vi "BatteryCharge1.vi"() -> ()   [LabVIEW 2020]
uses:
  <instrlib>/NH Research Regenerative Test Series/Public/Configure/Output Safety.ctl
  <instrlib>/NH Research Regenerative Test Series/Public/Data/Read (Ave Current).vi
  <instrlib>/NH Research Regenerative Test Series/Public/Data/Low Level/Fetch (Ave Voltage).vi
  <instrlib>/NH Research Regenerative Test Series/Public/Data/Low Level/Fetch (Ave True Power).vi
  <instrlib>/NH Research Regenerative Test Series/NH Research Regenerative Test Series.lvlib
panel:
  in  "Output Safety":T1
  out "Current Compare":dbl
  in  "Current Cutoff":dbl
  out "Ave Current (A)":dbl
  out "Ave Voltage (V)":dbl
  out "Ave True Power (W)":dbl
  out "Status Byte Register":T2
  in  "Logical Instrument Number":u32=1
  in  "Charge Current":dbl format="%#.6g"
  in  "Charge Voltage":dbl format="%#.6g"
  in  "Battery Detect Voltage (0V)":dbl format="%#.6g"
  in  "VISA resource name":refnum<visa-resource-name>
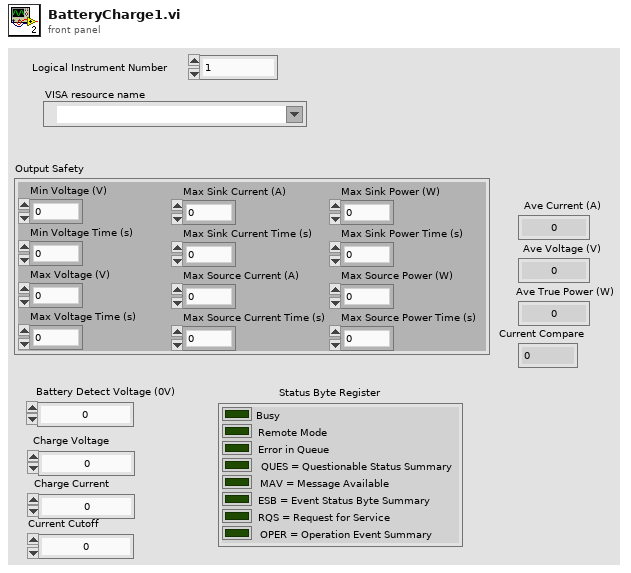
[diagram p1: front panel]
types:
  T1 = typedef "NH Research Regenerative Test Series.lvlib/Output Safety.ctl" = cluster{"Min Voltage (V)":dbl, "Min Voltage Time (s)":dbl, "Max Voltage (V)":dbl, "Max Voltage Time (s)":dbl, "Max Sink Current (A)":dbl, "Max Sink Current Time (s)":dbl, "Max Source Current (A)":dbl, "Max Source Current Time (s)":dbl, "Max Sink Power (W)":dbl, "Max Sink Power Time (s)":dbl, "Max Source Power (W)":dbl, "Max Source Power Time (s)":dbl}
  T2 = cluster{"Busy":bool, "Remote Mode":bool, "Error in Queue":bool, "QUES = Questionable Status Summary":bool, "MAV = Message Available":bool, "ESB = Event Status Byte Summary":bool, "RQS = Request for Service":bool, "OPER = Operation Event Summary":bool}
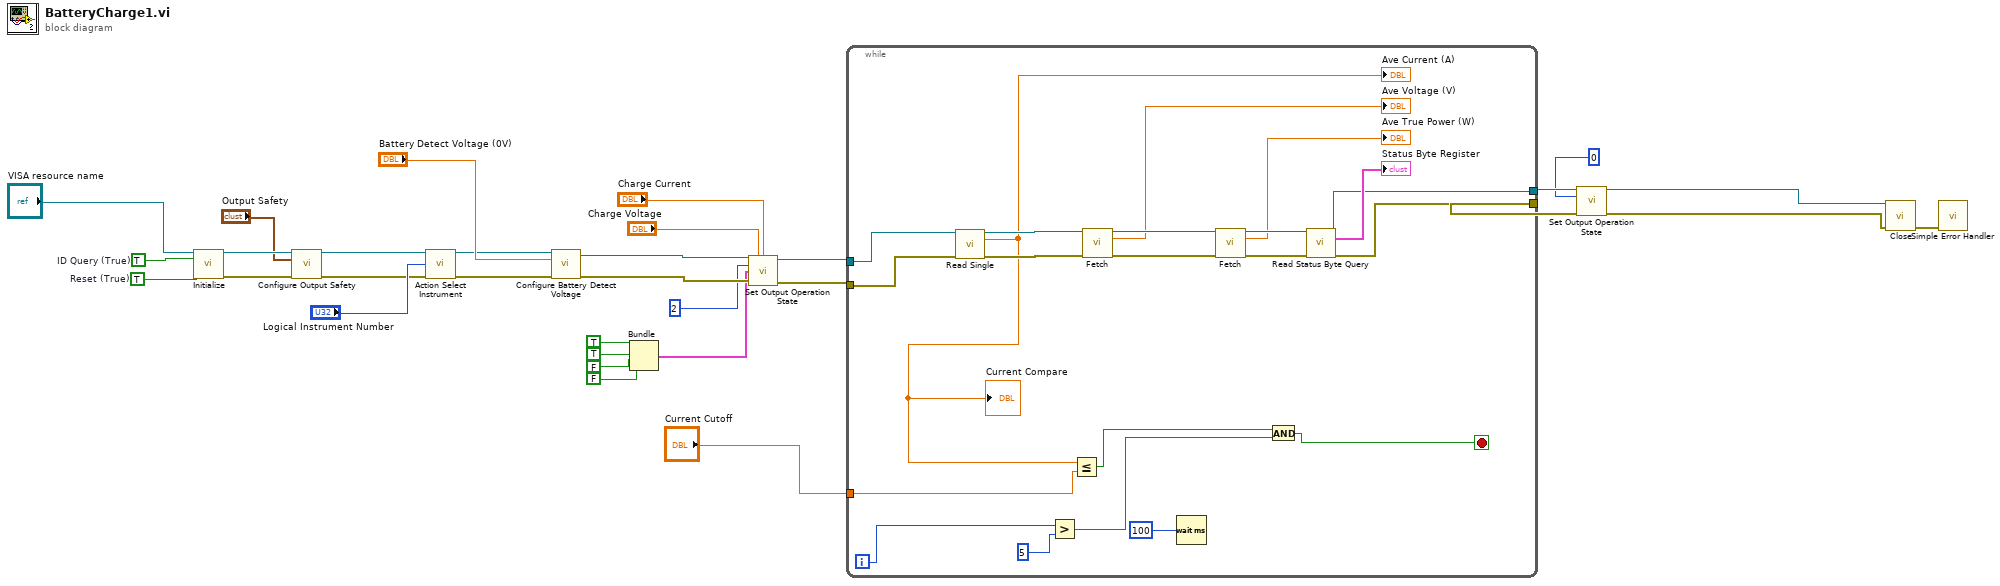
[diagram p0: block diagram]
diagram:
  w11 = TRUE  # ID Query (True)
  w10 = TRUE  # Reset (True)
  n1 = call <vilib>:"Initialize.vi"("VISA resource name"="VISA resource name", "ID Query (True)"=w11, "Reset (True)"=w10) -> ("VISA resource name out"=w9:refnum<visa-resource-name>, "error out"=w8:errorcluster)  [unwired: 11 in]
  n2 = call <vilib>:"Configure Output Safety.vi"("VISA resource name"=w9, "Output Safety"="Output Safety", "error in (no error)"=w8) -> ("VISA resource name out"=w5:refnum<visa-resource-name>, "error out"=w1:errorcluster)  [unwired: 11 in]
  n3 = call <instrlib>:"Action Select Instrument.vi"("VISA resource name"=w5, "Logical Instrument Number"="Logical Instrument Number", "error in (no error)"=w1) -> ("VISA resource name out"=w28:refnum<visa-resource-name>, "error out"=w27:errorcluster)  [unwired: 11 in]
  n4 = call <vilib>:"Configure Battery Detect Voltage.vi"("VISA resource name"=w28, "Battery Detect Voltage (0V)"="Battery Detect Voltage (0V)", "error in (no error)"=w27) -> ("VISA resource name out"=w26:refnum<visa-resource-name>, "error out"=w25:errorcluster)  [unwired: 11 in]
  n5 = Bundle(TRUE, TRUE, FALSE, FALSE) -> (w13:cluster{bool, bool, bool, bool})  [unwired: 1 in]
  n6 = call <vilib>:"Set Output Operation State.vi"("VISA resource name"=w26, "Voltage Setpoint (0 V)"="Charge Voltage", "Current Setpoint (0 A)"="Charge Current", "Mode (0: Off)"=2, "Enable"=w13, "error in (no error)"=w25) -> ("VISA resource name out"=w21:refnum<visa-resource-name>, "error out"=w20:errorcluster)  [unwired: 8 in]
  n7 = while {
    tunnel: w21 -> [w46]
    tunnel: w20 -> [w45]
    tunnel: [w43] -> w24
    tunnel: [w42] -> w23
    tunnel: "Current Cutoff" -> [w40]
    i -> [w36]
    stop <- w32 stop-if-true
    n8 = call-poly <instrlib>:"Read Single.vi"("VISA resource name"=w46, "error in (no error)"=w45) -> ("VISA resource name out"=w51:refnum<visa-resource-name>, "Ave Current (A)"=w38:dbl, "error out"=w52:errorcluster)  [unwired: 11 in]
    "Ave Current (A)" <- w38
    "Current Compare" <- w38
    n9 = Greater?(x=w36, y=5) -> (0:w34:bool)
    n10 = Less Or Equal?(x=w38, y=w40) -> (x <= y?=w33:bool)
    n11 = call-poly <instrlib>:"Fetch.vi"("VISA resource name"=w51, "error in (no error)"=w52) -> ("VISA resource name out"=w50:refnum<visa-resource-name>, "Ave Voltage (V)"=→"Ave Voltage (V)":dbl, "error out"=w49:errorcluster)  [unwired: 11 in]
    n12 = Wait (ms)(milliseconds to wait=100) -> ()  [unwired: 1 out]
    n13 = call-poly <instrlib>:"Fetch.vi"("VISA resource name"=w50, "error in (no error)"=w49) -> ("VISA resource name out"=w48:refnum<visa-resource-name>, "Ave True Power (W)"=→"Ave True Power (W)":dbl, "error out"=w47:errorcluster)  [unwired: 11 in]
    n14 = And(x=w33, y=w34) -> (x .and. y?=w32:bool)
    n15 = call <instrlib>:"Read Status Byte Query.vi"("VISA resource name"=w48, "error in (no error)"=w47) -> ("VISA resource name out"=w43:refnum<visa-resource-name>, "Status Byte Register"=→"Status Byte Register":T2, "error out"=w42:errorcluster)  [unwired: 11 in]
  }
  n16 = call <vilib>:"Set Output Operation State.vi"("VISA resource name"=w24, "Mode (0: Off)"=0, "error in (no error)"=w23) -> ("VISA resource name out"=w3:refnum<visa-resource-name>, "error out"=w2:errorcluster)  [unwired: 11 in]
  n17 = call <instrlib>:"Close.vi"("VISA resource name"=w3, "error in (no error)"=w2) -> ("error out"=w4:errorcluster)  [unwired: 13 in]
  n18 = call <vilib>:"Simple Error Handler.vi"("error in (no error)"=w4) -> ()  [unwired: 4 in, 5 out]
